vi "AddControl.vi"(6 "Attrs in":T1, 7 "Ctrl in":u32, 8 "error in":errorcluster, 9 "delay in":u32, 10 "Attrs array in":T1[](array[typedef]), 11 "Ctrl array in":u32[](array[numeric])) -> (0 "error out":errorcluster, 1 "delay out":u32, 2 "Attrs array out":T1[](array[typedef]), 3 "Ctrl array out":u32[](array[numeric]))   [LabVIEW 2012, in "Spinner.xctl"]
uses:
  Spinner.xctl
  Attrs.ctl
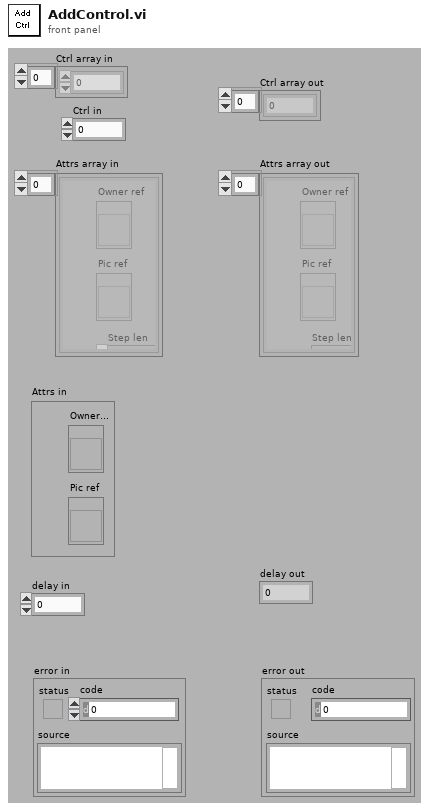
[diagram p1: front panel]
types:
  T1 = typedef "Spinner.xctl/Attrs.ctl" = cluster{"Owner ref":refnum<vi>, "Pic ref":refnum<vi>, "Step len":dbl, "Imgs":picture[], "Current phase":dbl}
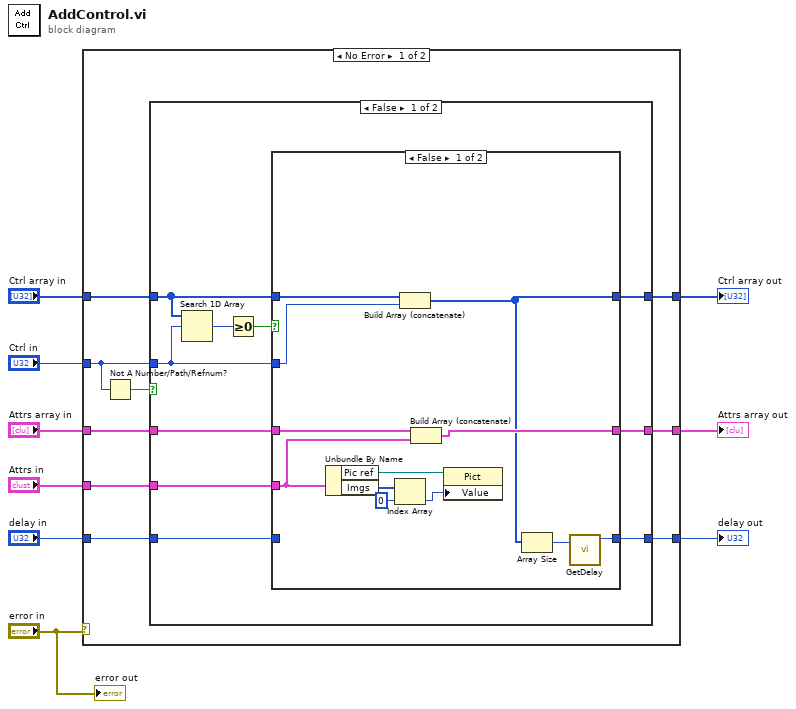
[diagram p0: block diagram]
diagram:
  n1 = case shown="No Error" "error in" {
    tunnel: "Ctrl in" -> [w16 _]
    tunnel: "Ctrl array in" -> [w17 w49]
    tunnel: "Attrs array in" -> [w15 w48]
    tunnel: "Attrs in" -> [w14 _]
    tunnel: [w13 w48] -> w5
    tunnel: [w12 w49] -> w4
    tunnel: [w11 w47] -> w3
    tunnel: "delay in" -> [w10 w47]
    frame No Error {
      n2 = Not A Number/Path/Refnum?(number/path/refnum=w16) -> (NaN/Path/Refnum?=w18:bool)
      n3 = case shown="False" w18 {
        tunnel: w17 -> [w23 w46]
        tunnel: w16 -> [w22 _]
        tunnel: w15 -> [w27 w45]
        tunnel: w14 -> [w25 _]
        tunnel: [w24 w45] -> w13
        tunnel: [w21 w46] -> w12
        tunnel: [w20 w44] -> w11
        tunnel: w10 -> [w19 w44]
        frame False {
          n4 = Search 1D Array(1D array=w23, element=w22) -> (index of element=w26:i32)  [unwired: 1 in]
          n5 = Greater Or Equal To 0?(x=w26) -> (x >= 0?=w28:bool)
          n6 = case shown="False" w28 {
            tunnel: w27 -> [w40 w42]
            tunnel: w25 -> [w33 _]
            tunnel: [w39 w42] -> w24
            tunnel: w23 -> [w38 w43]
            tunnel: w22 -> [w37 _]
            tunnel: [w35 w43] -> w21
            tunnel: [w34 w41] -> w20
            tunnel: w19 -> [_ w41]
            frame False {
              n7 = Unbundle By Name(w33) -> ("Pic ref"=w30:refnum<vi>, "Imgs"=w32:picture[])
              n8 = Index Array(array=w32, index=0) -> (element=w29:picture)
              n9 = Build Array (concatenate)(w38, w37) -> (w35:u32[])
              n10 = Build Array (concatenate)(w40, w33) -> (w39:T1[])
              n11 = property class="Pict"(reference=w30, "Value"=w29) -> ()  [unwired: 1 in, 2 out]
              n12 = Array Size(array=w35) -> (size(s)=w36:i32)
              n13 = call "GetDelay.vi"("Count"=w36) -> ("Delay"=w34:u32)  [unwired: 9 in, 1 out]
            }
            frame True {
            }
          }
        }
        frame True {
        }
      }
    }
    frame Error {
    }
  }
  "Attrs array out" <- w5
  "Ctrl array out" <- w4
  "delay out" <- w3
  "error out" <- "error in"
